vi "S2DS_Data Save Info.vi"(0 "User info":string[](array[string]), 1 "All channel info (in)":T1={"WCl names with units"=[], "RC  names with units"=[], "DC  names with units"=[""], "AC names with units"=[], "Indicator captions"=[], "Graph channels"=[], "Channel numbers"=[], "User info"=""}, 2 "False channels":string[][](array[string])) -> (7 "Data save info (out)":T2={"File path"=path "", "Header"="", "File name"="", "False channel"=[], "Channel names"=[], "Buffer size"=0, "Format"="%.6f"})   [LabVIEW 2025]
uses:
  TYPE DEFS/S2DS_Data saving info.ctl
  TYPE DEFS/S2DS_Display info.ctl
  <vilib>/Utility/sysdir.llb/System Directory Type.ctl
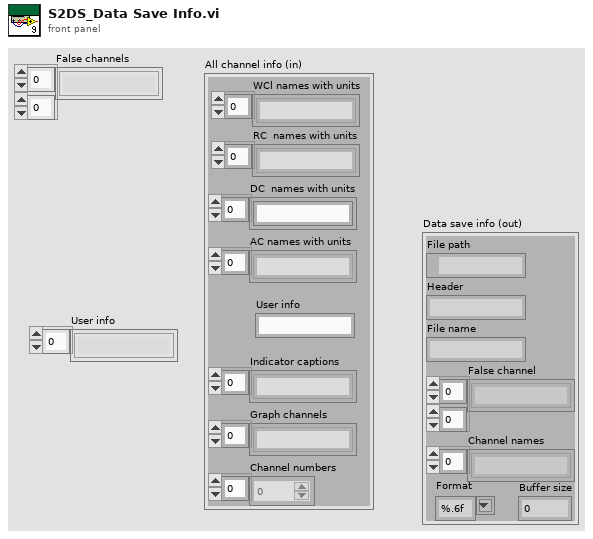
[diagram p1: front panel]
types:
  T1 = typedef "S2DS_Display info.ctl" = cluster{"WCl names with units":string[], "RC  names with units":string[], "DC  names with units":string[], "AC names with units":string[], "Indicator captions":string[], "Graph channels":string[], "Channel numbers":i32[], "User info":string}
  T2 = typedef "S2DS_Data saving info.ctl" = cluster{"File path":path, "Header":string, "File name":string, "False channel":string[][], "Channel names":string[], "Buffer size":i32, "Format":string}
  T3 = typedef "System Directory Type.ctl" = i32
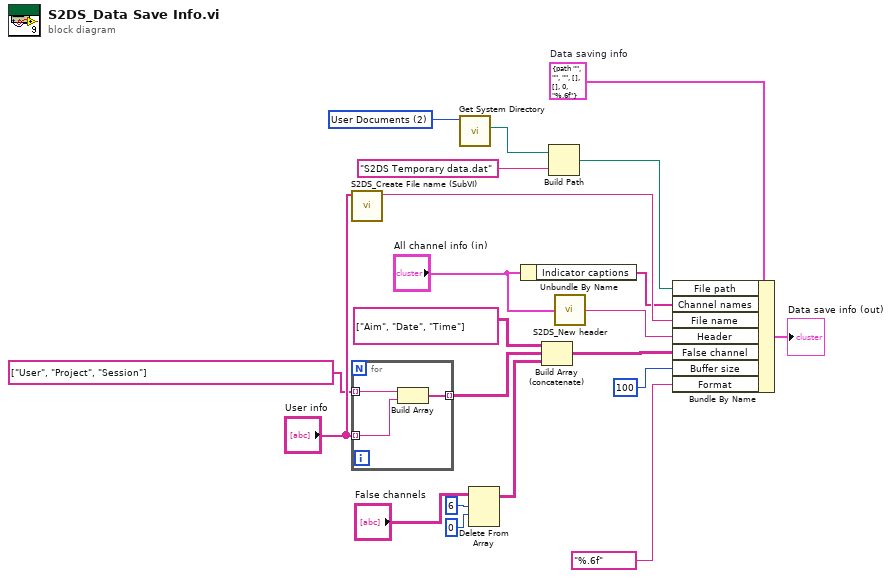
[diagram p0: block diagram]
diagram:
  w16 = T3 2 items=["User Home"=0, "User Desktop"=1, "User Documents"=2, "User Application Data"=3, "User Preferences"=4, "User Temporary"=5, "Public Documents"=6, "Public Application Data"=7, "Public Preferences"=8, "Public Cache"=13, "System Core Libraries"=9, "System Installed Libraries"=10, "Application Files"=11, "Boot Volume Root"=12] ("system directory type")
  w13 = T2 {"File path"=path "", "Header"="", "File name"="", "False channel"=[], "Channel names"=[], "Buffer size"=0, "Format"="%.6f"}  # Data saving info
  n1 = call "S2DS_Create File name (SubVI).vi"("User info"="User info") -> ("File name"=w21:string)  [unwired: 10 in]
  n2 = for {
    tunnel: "User info" -> [w22] mode=indexing
    tunnel: string[] ["User", "Project", "Session"] -> [w23] mode=indexing
    tunnel: [w24] -> w8 mode=indexing
    n3 = Build Array(w23, w22) -> (w24:string[])
  }
  n4 = call <vilib>:"Get System Directory.vi"("system directory type"=w16) -> ("system directory"=w15:path)  [unwired: 10 in]
  n5 = Delete From Array(array="False channels", length=6, index (row)=0) -> (array with subset deleted=w1:string[][])  [unwired: 1 in, 1 out]
  n6 = Unbundle By Name("All channel info (in)") -> ("Indicator captions"=w9:string[])
  n7 = Build Array (concatenate)(string[][] [["Aim"], ["Date"], ["Time"]], w8, w1) -> (w17:string[][])
  n8 = Build Path(base path=w15, name or relative path="S2DS Temporary data.dat") -> (appended path=w12:path)
  n9 = call "S2DS_New header.vi"("Complete channel name info"="All channel info (in)") -> ("Header (out)"=w20:string)  [unwired: 2 in]
  n10 = Bundle By Name(cluster=w13, "File path"=w12, "Channel names"=w9, "File name"=w21, "Header"=w20, "False channel"=w17, "Buffer size"=100, "Format"="%.6f") -> (→"Data save info (out)":T2)
